vi "Collect Data.vi"(8 "error in (no error)":errorcluster, 10 "AbstractData in":refnum<class "AbstractData.lvclass">, 11 "AbstractCollector in":refnum<class "AbstractCollector.lvclass">) -> (0 "error out":errorcluster, 2 "finished?":bool=TRUE, 3 "AbstractCollector out":refnum<class "AbstractCollector.lvclass">)   [LabVIEW 2014, in "AbstractCollector.lvclass"]
uses:
  AbstractCollector.lvclass
  Model/Data/AbstractData/AbstractData.lvclass
  AbstractCollector.lvclass/AbstractCollector.ctl
  Interfaces/Observable Actor/Observable Actor.lvclass
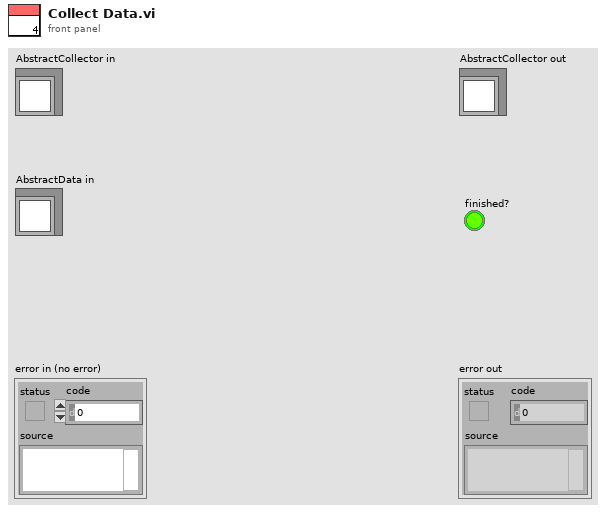
[diagram p1: front panel]
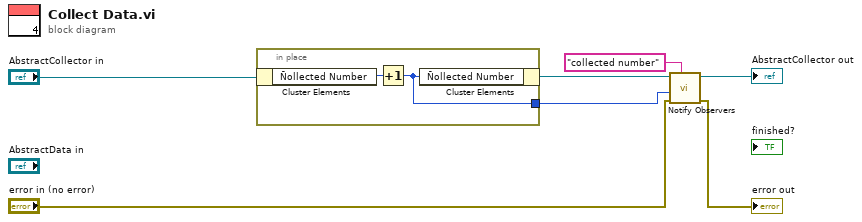
[diagram p0: block diagram]
diagram:
  n1 = in-place {
    in-place-border: [w8] -> w2
    n2 = in-place-cluster #1("AbstractCollector in") -> ("Ñollected Number"=w9:u32)
    n3 = Increment(x=w9) -> (x+1=w8:u32)
    n4 = in-place-cluster #1("Ñollected Number"=w8) -> (w3:refnum<class "AbstractCollector.lvclass">)
  }
  n5 = call "Notify Observers.vi"("name"="collected number", "error in (no error)"="error in (no error)", "value"=w2, "Observable Actor in"=w3) -> ("error out"=→"error out":errorcluster, "Observable Actor out"=→"AbstractCollector out":refnum<class "AbstractCollector.lvclass">)  [unwired: 6 in]
